vi "AUTON_Index.vi"(0 "Auton Array":dbl[][](array[numeric]), 5 "MeasuredHeading":dbl, 7 "LeftEncoder":dbl, 9 "RightEncoder":dbl) -> (4 "Right Drive":dbl, 6 "Left Drive":dbl, 8 "Harvester":dbl, 10 "Winch":dbl, 14 "Roller":dbl, 15 "Cam":dbl)   [LabVIEW 2013]
uses:
  Robot Global Data.vi
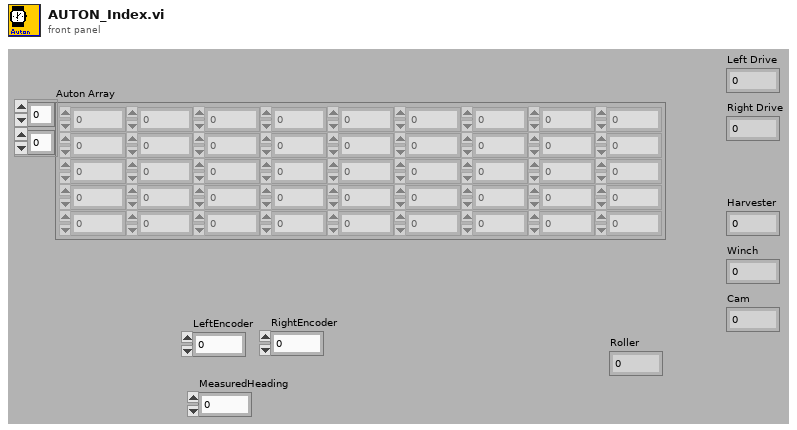
[diagram p1: front panel]
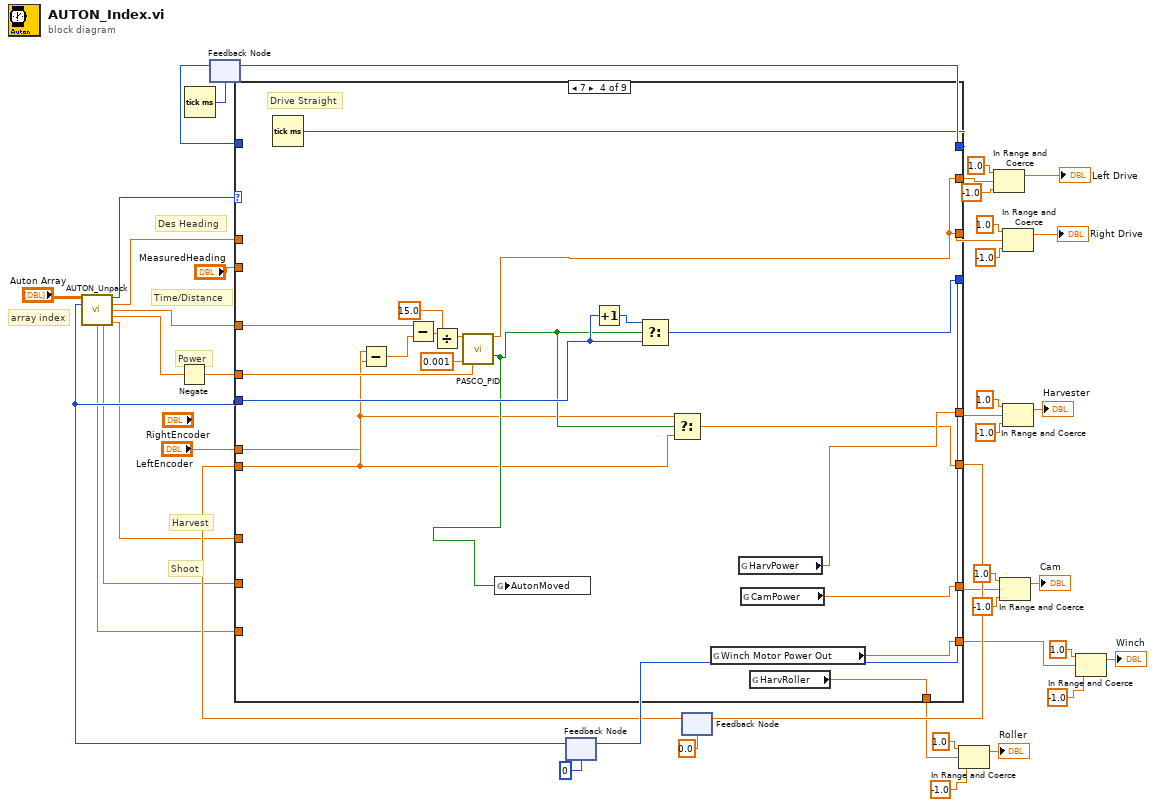
[diagram p0: block diagram]
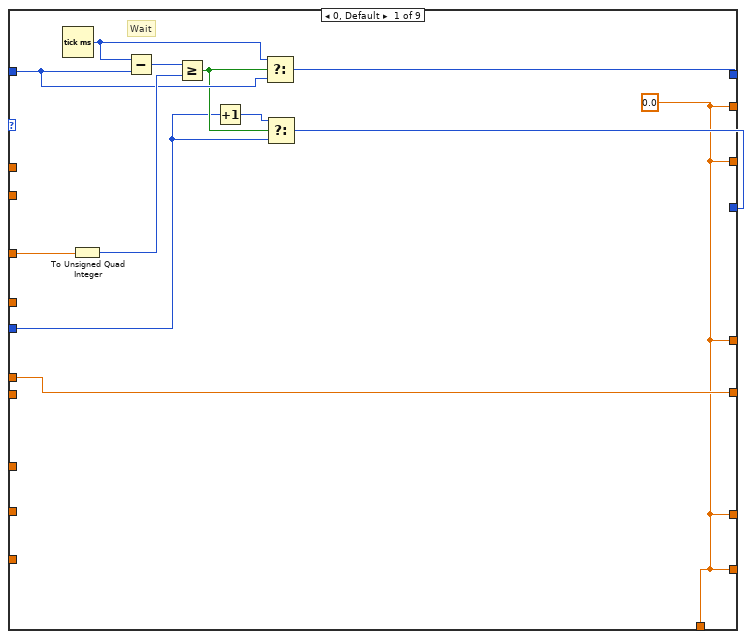
[diagram p2: hidden frame]
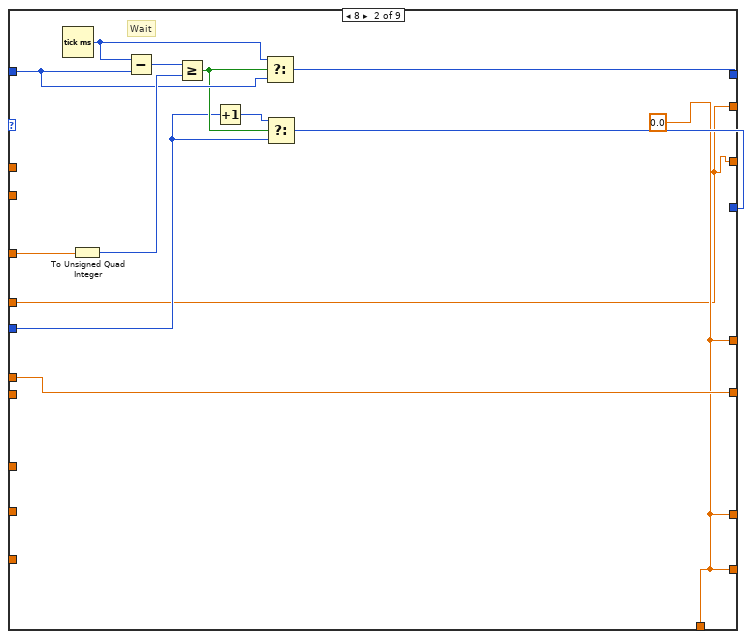
[diagram p3: hidden frame]
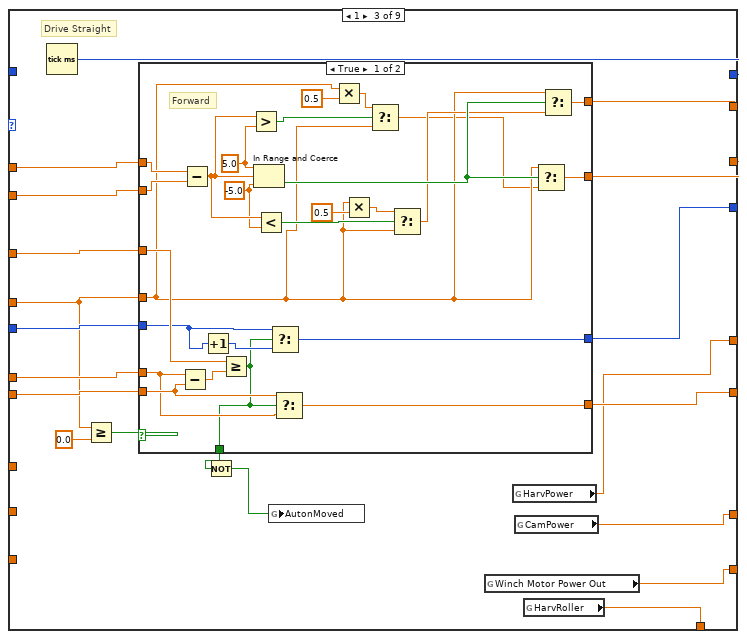
[diagram p4: hidden frame]
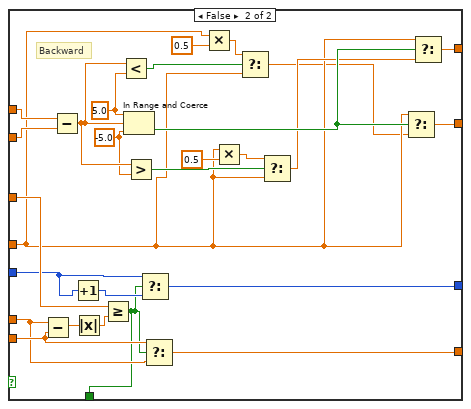
[diagram p5: hidden frame]
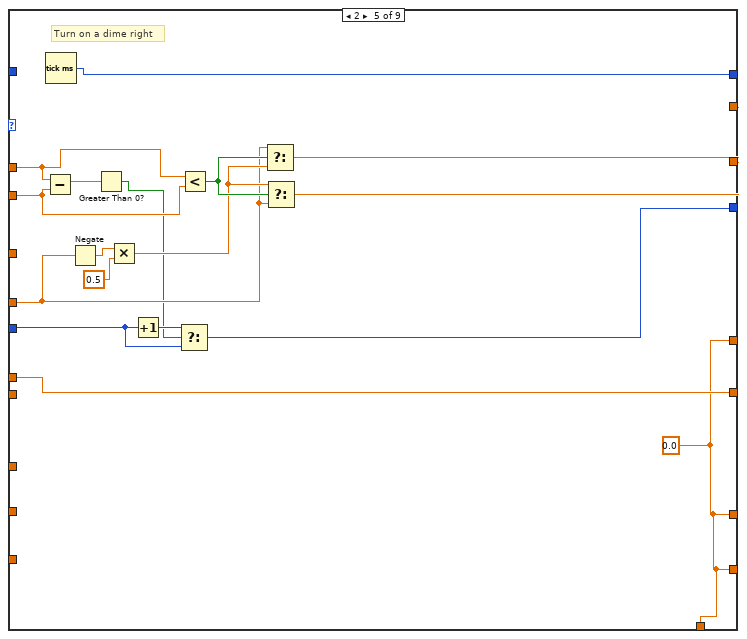
[diagram p6: hidden frame]
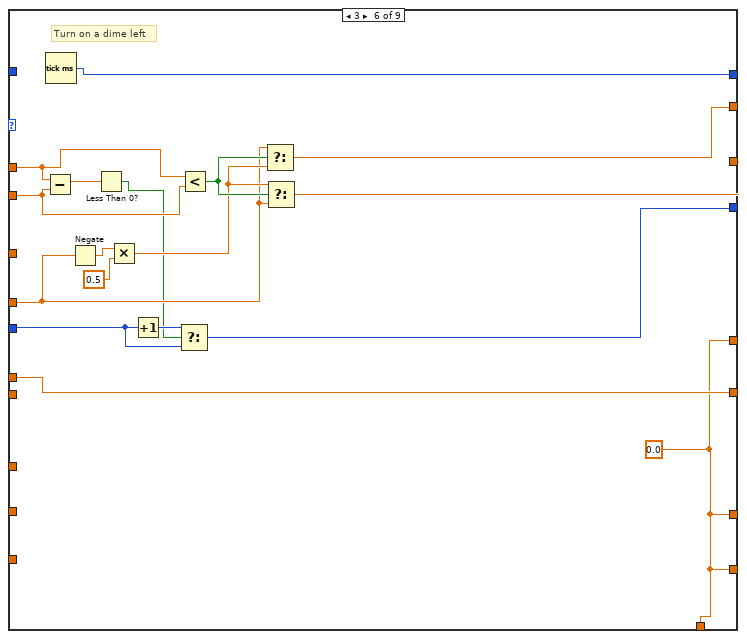
[diagram p7: hidden frame]
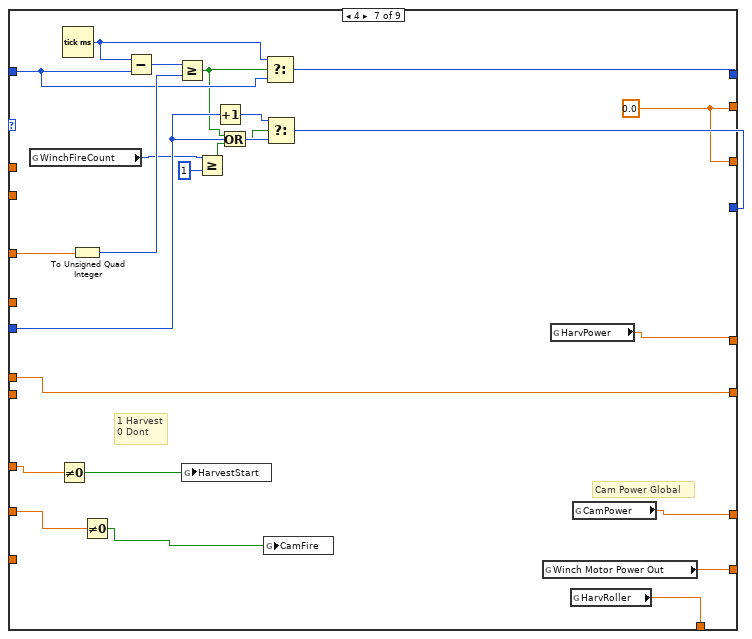
[diagram p8: hidden frame]
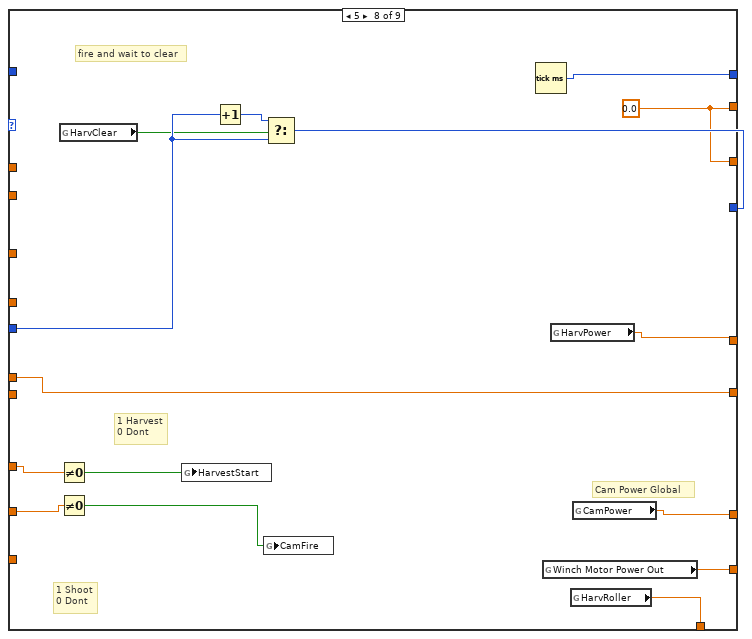
[diagram p9: hidden frame]
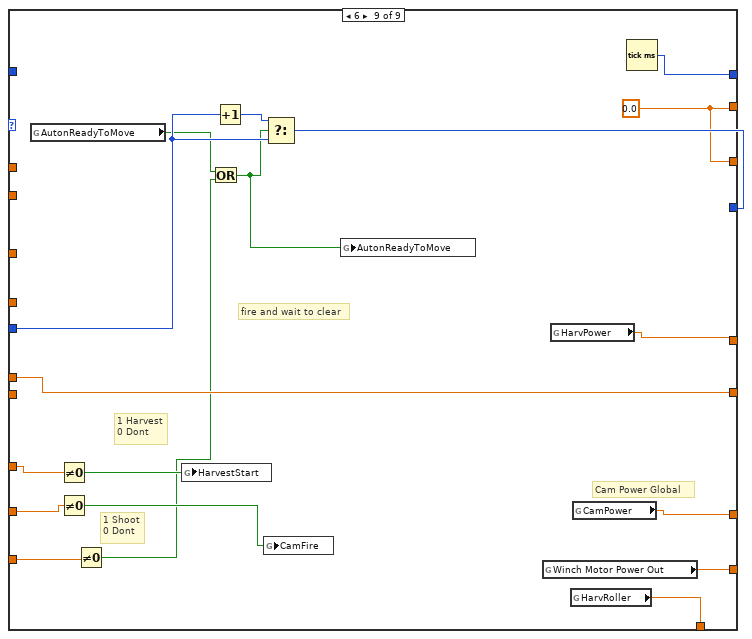
[diagram p10: hidden frame]
diagram:
  # "Shoot"
  # "Harvest"
  # "Des Heading"
  # "Time/Distance"
  # "Power"
  # "array index"
  n1 = Tick Count (ms)() -> (millisecond timer value=w42:u32)
  n2 = feedback #1(w42) -> (w43:u32)
  n3 = feedback #2(0) -> (w23:i32)
  n4 = call "AUTON_Unpack.vi"("all rows"="Auton Array", "Index"=w23) -> ("Primitive ID"=w26:i16, "Desired Heading"=w25:dbl, "Time/Distance"=w24:dbl, "Power"=w11:dbl, "Moved"=w1:dbl, "Shoot"=w8:dbl, "Harvest"=w9:dbl)  [unwired: 7 in]
  n5 = Negate(x=w11) -> (-x=w10:dbl)
  n6 = feedback #3(0.0) -> (w28:dbl)
  n7 = case shown="7" w26 {
    tunnel: [w48 w61 w87 w156 w174 w191 w213 w233 w251] -> w30
    tunnel: w23 -> [w49 w62 w82 w154 w177 w194 w214 w234 w252]
    tunnel: [w56 w69 w79 w162 w179 w196 w220 w224 w240] -> w32
    tunnel: w43 -> [w53 w66 _ _ _ _ w217 _ _]
    tunnel: w24 -> [w47 w60 w88 w146 _ _ w212 _ _]
    tunnel: w25 -> [_ _ w86 _ w172 w189 _ _ _]
    tunnel: [w45 w57 w84 w144 w175 w192 w211 w232 w250] -> w40
    tunnel: [w45 w57 w83 w144 w176 w193 w211 w232 w250] -> w33
    tunnel: w10 -> [_ w57 w78 w157 w166 w183 _ _ _]
    tunnel: "LeftEncoder" -> [w46 w59 w80 w149 w173 w190 w210 w231 w249]
    tunnel: "MeasuredHeading" -> [_ _ w85 _ w171 w188 _ _ _]
    tunnel: w28 -> [_ _ w81 w150 _ _ _ _ _]
    tunnel: [w46 w59 w89 w152 w173 w190 w210 w231 w249] -> w27
    tunnel: [w45 w58 w75 w161 w163 w180 w208 w229 w247] -> w13
    tunnel: [w45 w58 w73 w159 w163 w180 w209 w230 w248] -> w12
    tunnel: w9 -> [_ _ _ _ _ _ w205 w227 w245]
    tunnel: w8 -> [_ _ _ _ _ _ w207 w222 w242]
    tunnel: [w45 w58 w74 w160 w163 w180 w206 w228 w246] -> w7
    tunnel: [w45 w58 w72 w158 w163 w180 w202 w225 w243] -> w3
    tunnel: w1 -> [_ _ _ _ _ _ _ _ w239]
    frame 0, Default {
      w45 = 0.0 ("Numeric")
      # "Wait"
      n8 = Tick Count (ms)() -> (millisecond timer value=w52:u32)
      n9 = To Unsigned Quad Integer(1:w47) -> (0:w54:u64)
      n10 = Subtract(x=w52, y=w53) -> (x-y=w55:u32)
      n11 = Greater Or Equal?(x=w55, y=w54) -> (x >= y?=w51:bool)
      n12 = Increment(x=w49) -> (x+1=w50:i32)
      n13 = Select(t=w52, s=w51, f=w53) -> (s? t:f=w56:u32)
      n14 = Select(t=w50, s=w51, f=w49) -> (s? t:f=w48:i32)
    }
    frame 8 {
      w58 = 0.0 ("Numeric")
      # "Wait"
      n15 = Tick Count (ms)() -> (millisecond timer value=w65:u32)
      n16 = To Unsigned Quad Integer(1:w60) -> (0:w67:u64)
      n17 = Subtract(x=w65, y=w66) -> (x-y=w68:u32)
      n18 = Greater Or Equal?(x=w68, y=w67) -> (x >= y?=w64:bool)
      n19 = Increment(x=w62) -> (x+1=w63:i32)
      n20 = Select(t=w65, s=w64, f=w66) -> (s? t:f=w69:u32)
      n21 = Select(t=w63, s=w64, f=w62) -> (s? t:f=w61:i32)
    }
    frame 1 {
      # "Drive Straight"
      n22 = Tick Count (ms)() -> (millisecond timer value=w79:u32)
      n23 = Greater Or Equal?(x=w78, y=0.0) -> (x >= y?=w76:bool)
      n24 = case shown="True" w76 {
        tunnel: [w115 w142] -> w89
        tunnel: w88 -> [w113 w141]
        tunnel: [w112 w140] -> w87
        tunnel: w86 -> [w111 w139]
        tunnel: w85 -> [w110 w138]
        tunnel: [w108 w136] -> w84
        tunnel: [w107 w135] -> w83
        tunnel: w78 -> [w96 w124]
        tunnel: w82 -> [w93 w121]
        tunnel: w81 -> [w92 w120]
        tunnel: w80 -> [w91 w119]
        tunnel: [w90 w116] -> w71
        frame True {
          w104 = -5.0 ("lower limit")
          w106 = 5.0 ("upper limit")
          # "Forward"
          n25 = Subtract(x=w91, y=w92) -> (x-y=w114:dbl)
          n26 = Subtract(x=w111, y=w110) -> (x-y=w105:dbl)
          n27 = Increment(x=w93) -> (x+1=w94:i32)
          n28 = Greater Or Equal?(x=w113, y=w114) -> (x >= y?=w90:bool)
          n29 = Greater?(x=w105, y=w106) -> (0:w99:bool)
          n30 = In Range and Coerce(upper limit=w106, x=w105, lower limit=w104) -> (In Range?=w109:bool)  [unwired: 1 out]
          n31 = Less?(x=w105, y=w104) -> (x < y?=w103:bool)
          n32 = Select(t=w93, s=w90, f=w94) -> (s? t:f=w112:i32)
          n33 = Select(t=w92, s=w90, f=w91) -> (s? t:f=w115:dbl)
          n34 = Multiply(x=w96, y=0.5) -> (x*y=w98:dbl)
          n35 = Multiply(x=w96, y=0.5) -> (x*y=w101:dbl)
          n36 = Select(t=w98, s=w99, f=w96) -> (s? t:f=w95:dbl)
          n37 = Select(t=w101, s=w103, f=w96) -> (s? t:f=w100:dbl)
          n38 = Select(t=w96, s=w109, f=w95) -> (s? t:f=w107:dbl)
          n39 = Select(t=w96, s=w109, f=w100) -> (s? t:f=w108:dbl)
        }
        frame False {
          w132 = -5.0 ("lower limit")
          w134 = 5.0 ("upper limit")
          # "Backward"
          n40 = Subtract(x=w119, y=w120) -> (x-y=w117:dbl)
          n41 = Subtract(x=w139, y=w138) -> (x-y=w133:dbl)
          n42 = Increment(x=w121) -> (x+1=w122:i32)
          n43 = Absolute Value(x=w117) -> (abs(x)=w118:dbl)
          n44 = Greater Or Equal?(x=w141, y=w118) -> (x >= y?=w116:bool)
          n45 = Less?(x=w133, y=w134) -> (x < y?=w127:bool)
          n46 = In Range and Coerce(upper limit=w134, x=w133, lower limit=w132) -> (In Range?=w137:bool)  [unwired: 1 out]
          n47 = Greater?(x=w133, y=w132) -> (0:w131:bool)
          n48 = Select(t=w121, s=w116, f=w122) -> (s? t:f=w140:i32)
          n49 = Select(t=w120, s=w116, f=w119) -> (s? t:f=w142:dbl)
          n50 = Multiply(x=w124, y=0.5) -> (x*y=w126:dbl)
          n51 = Multiply(x=w124, y=0.5) -> (x*y=w129:dbl)
          n52 = Select(t=w126, s=w127, f=w124) -> (s? t:f=w123:dbl)
          n53 = Select(t=w129, s=w131, f=w124) -> (s? t:f=w128:dbl)
          n54 = Select(t=w124, s=w137, f=w123) -> (s? t:f=w135:dbl)
          n55 = Select(t=w124, s=w137, f=w128) -> (s? t:f=w136:dbl)
        }
      }
      n56 = Not(x=w71) -> (.not. x?=w70:bool)
      n57 = global write "Robot Global Data.vi" "AutonMoved"(w70) -> ()
      n58 = global read "Robot Global Data.vi" "Winch Motor Power Out"() -> (w74:dbl)
      n59 = global read "Robot Global Data.vi" "HarvPower"() -> (w73:dbl)
      n60 = global read "Robot Global Data.vi" "CamPower"() -> (w75:dbl)
      n61 = global read "Robot Global Data.vi" "HarvRoller"() -> (w72:dbl)
    }
    frame 7 {
      # "Drive Straight"
      n62 = Tick Count (ms)() -> (millisecond timer value=w162:u32)
      n63 = Subtract(x=w150, y=w149) -> (x-y=w151:dbl)
      n64 = Subtract(x=w146, y=w151) -> (x-y=w147:dbl)
      n65 = Divide(x=w147, y=15.0) -> (x/y=w148:dbl)
      n66 = call "PASCO_PID.vi"("Delta"=w148, "Deadband"=0.001, "P Gain"=w157) -> ("Output"=w144:dbl, "IsThere"=w153:bool)  [unwired: 11 in]
      n67 = global write "Robot Global Data.vi" "AutonMoved"(w153) -> ()
      n68 = Increment(x=w154) -> (x+1=w155:i32)
      n69 = Select(t=w155, s=w153, f=w154) -> (s? t:f=w156:i32)
      n70 = Select(t=w149, s=w153, f=w150) -> (s? t:f=w152:dbl)
      n71 = global read "Robot Global Data.vi" "Winch Motor Power Out"() -> (w160:dbl)
      n72 = global read "Robot Global Data.vi" "HarvPower"() -> (w159:dbl)
      n73 = global read "Robot Global Data.vi" "CamPower"() -> (w161:dbl)
      n74 = global read "Robot Global Data.vi" "HarvRoller"() -> (w158:dbl)
    }
    frame 2 {
      w163 = 0.0 ("Numeric")
      # "Turn on a dime right"
      n75 = Subtract(x=w172, y=w171) -> (x-y=w165:dbl)
      n76 = Tick Count (ms)() -> (millisecond timer value=w179:u32)
      n77 = Negate(x=w166) -> (-x=w169:dbl)
      n78 = Greater Than 0?(x=w165) -> (x > 0?=w164:bool)
      n79 = Multiply(x=w169, y=0.5) -> (x*y=w167:dbl)
      n80 = Increment(x=w177) -> (x+1=w178:i32)
      n81 = Select(t=w178, s=w164, f=w177) -> (s? t:f=w174:i32)
      n82 = Less?(x=w172, y=w171) -> (x < y?=w170:bool)
      n83 = Select(t=w166, s=w170, f=w167) -> (s? t:f=w175:dbl)
      n84 = Select(t=w167, s=w170, f=w166) -> (s? t:f=w176:dbl)
    }
    frame 3 {
      w180 = 0.0 ("Numeric")
      # "Turn on a dime left"
      n85 = Subtract(x=w189, y=w188) -> (x-y=w182:dbl)
      n86 = Tick Count (ms)() -> (millisecond timer value=w196:u32)
      n87 = Negate(x=w183) -> (-x=w186:dbl)
      n88 = Less Than 0?(x=w182) -> (x < 0?=w181:bool)
      n89 = Multiply(x=w186, y=0.5) -> (x*y=w184:dbl)
      n90 = Increment(x=w194) -> (x+1=w195:i32)
      n91 = Select(t=w195, s=w181, f=w194) -> (s? t:f=w191:i32)
      n92 = Less?(x=w189, y=w188) -> (x < y?=w187:bool)
      n93 = Select(t=w183, s=w187, f=w184) -> (s? t:f=w192:dbl)
      n94 = Select(t=w184, s=w187, f=w183) -> (s? t:f=w193:dbl)
    }
    frame 4 {
      w211 = 0.0 ("Numeric")
      # "1 Harvest\n0 Dont"
      # "Cam Power Global"
      n95 = global read "Robot Global Data.vi" "WinchFireCount"() -> (w198:i32)
      n96 = Not Equal To 0?(x=w205) -> (x != 0?=w204:bool)
      n97 = Tick Count (ms)() -> (millisecond timer value=w216:u32)
      n98 = To Unsigned Quad Integer(1:w212) -> (0:w218:u64)
      n99 = Not Equal To 0?(x=w207) -> (x != 0?=w203:bool)
      n100 = Subtract(x=w216, y=w217) -> (x-y=w219:u32)
      n101 = Greater Or Equal?(x=w219, y=w218) -> (x >= y?=w200:bool)
      n102 = global write "Robot Global Data.vi" "HarvestStart"(w204) -> ()
      n103 = Greater Or Equal?(x=w198, y=1) -> (x >= y?=w199:bool)
      n104 = Increment(x=w214) -> (x+1=w215:i32)
      n105 = Or(x=w200, y=w199) -> (x .or. y?=w201:bool)
      n106 = global write "Robot Global Data.vi" "CamFire"(w203) -> ()
      n107 = Select(t=w216, s=w200, f=w217) -> (s? t:f=w220:u32)
      n108 = Select(t=w215, s=w201, f=w214) -> (s? t:f=w213:i32)
      n109 = global read "Robot Global Data.vi" "Winch Motor Power Out"() -> (w206:dbl)
      n110 = global read "Robot Global Data.vi" "HarvPower"() -> (w209:dbl)
      n111 = global read "Robot Global Data.vi" "HarvRoller"() -> (w202:dbl)
      n112 = global read "Robot Global Data.vi" "CamPower"() -> (w208:dbl)
    }
    frame 5 {
      w232 = 0.0 ("Numeric")
      # "fire and wait to clear"
      # "1 Harvest\n0 Dont"
      # "1 Shoot\n0 Dont"
      # "Cam Power Global"
      n113 = Not Equal To 0?(x=w227) -> (x != 0?=w226:bool)
      n114 = Not Equal To 0?(x=w222) -> (x != 0?=w221:bool)
      n115 = global read "Robot Global Data.vi" "HarvClear"() -> (w223:bool)
      n116 = global write "Robot Global Data.vi" "HarvestStart"(w226) -> ()
      n117 = Increment(x=w234) -> (x+1=w235:i32)
      n118 = global write "Robot Global Data.vi" "CamFire"(w221) -> ()
      n119 = Select(t=w235, s=w223, f=w234) -> (s? t:f=w233:i32)
      n120 = Tick Count (ms)() -> (millisecond timer value=w224:u32)
      n121 = global read "Robot Global Data.vi" "Winch Motor Power Out"() -> (w228:dbl)
      n122 = global read "Robot Global Data.vi" "HarvPower"() -> (w230:dbl)
      n123 = global read "Robot Global Data.vi" "HarvRoller"() -> (w225:dbl)
      n124 = global read "Robot Global Data.vi" "CamPower"() -> (w229:dbl)
    }
    frame 6 {
      w250 = 0.0 ("Numeric")
      # "fire and wait to clear"
      # "1 Harvest\n0 Dont"
      # "1 Shoot\n0 Dont"
      # "Cam Power Global"
      n125 = global read "Robot Global Data.vi" "AutonReadyToMove"() -> (w237:bool)
      n126 = Not Equal To 0?(x=w245) -> (x != 0?=w244:bool)
      n127 = Not Equal To 0?(x=w242) -> (x != 0?=w241:bool)
      n128 = Not Equal To 0?(x=w239) -> (x != 0?=w238:bool)
      n129 = global write "Robot Global Data.vi" "HarvestStart"(w244) -> ()
      n130 = Or(x=w237, y=w238) -> (x .or. y?=w236:bool)
      n131 = Increment(x=w252) -> (x+1=w253:i32)
      n132 = global write "Robot Global Data.vi" "CamFire"(w241) -> ()
      n133 = Select(t=w253, s=w236, f=w252) -> (s? t:f=w251:i32)
      n134 = global write "Robot Global Data.vi" "AutonReadyToMove"(w236) -> ()
      n135 = global read "Robot Global Data.vi" "Winch Motor Power Out"() -> (w246:dbl)
      n136 = global read "Robot Global Data.vi" "HarvPower"() -> (w248:dbl)
      n137 = global read "Robot Global Data.vi" "HarvRoller"() -> (w243:dbl)
      n138 = global read "Robot Global Data.vi" "CamPower"() -> (w247:dbl)
      n139 = Tick Count (ms)() -> (millisecond timer value=w240:u32)
    }
  }
  n140 = feedback-in #1(w32) -> ()
  n141 = feedback-in #2(w30) -> ()
  n142 = feedback-in #3(w27) -> ()
  n143 = In Range and Coerce(upper limit=1.0, x=w3, lower limit=-1.0) -> (coerced(x)=→"Roller":dbl)  [unwired: 1 out]
  n144 = In Range and Coerce(upper limit=1.0, x=w40, lower limit=-1.0) -> (coerced(x)=→"Left Drive":dbl)  [unwired: 1 out]
  n145 = In Range and Coerce(upper limit=1.0, x=w13, lower limit=-1.0) -> (coerced(x)=→"Cam":dbl)  [unwired: 1 out]
  n146 = In Range and Coerce(upper limit=1.0, x=w33, lower limit=-1.0) -> (coerced(x)=→"Right Drive":dbl)  [unwired: 1 out]
  n147 = In Range and Coerce(upper limit=1.0, x=w12, lower limit=-1.0) -> (coerced(x)=→"Harvester":dbl)  [unwired: 1 out]
  n148 = In Range and Coerce(upper limit=1.0, x=w7, lower limit=-1.0) -> (coerced(x)=→"Winch":dbl)  [unwired: 1 out]
